vi "Example Callback - CO2Concentration Callback.vi"(4 "CO2Concentration":refnum<user-event>, 5 "Event Data":T1, 6 "Control Ref":refnum<k24>, 7 "Event Common Data":T2) -> ()   [LabVIEW 2010]
uses:
  C:/tf/play/labview/Tinkerforge.dll
  Tinkerforge.dll
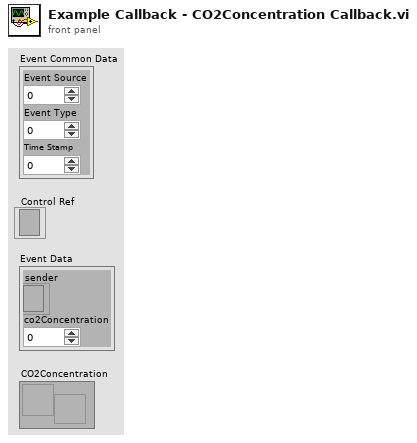
[diagram p1: front panel]
types:
  T1 = cluster{"sender":refnum<k24>, "co2Concentration":i32}
  T2 = cluster{"Event Source":i32, "Event Type":u32, "Time Stamp":u32}
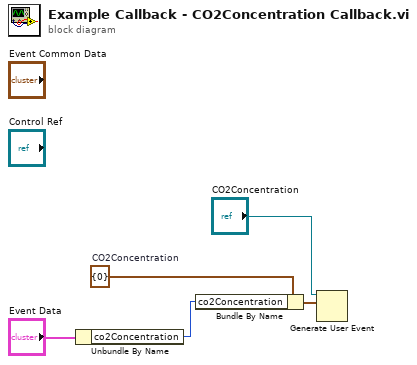
[diagram p0: block diagram]
diagram:
  w3 = cluster{"co2Concentration":i32} {"co2Concentration"=0}  # CO2Concentration
  n1 = Unbundle By Name("Event Data") -> ("co2Concentration"=w4:i32)
  n2 = Bundle By Name(cluster=w3, "co2Concentration"=w4) -> (w2:cluster{"co2Concentration":i32})
  n3 = Generate User Event(user event="CO2Concentration", event data cluster=w2) -> ()  [unwired: 1 in, 2 out]
